vi "Read FP Control.vi"(8 "error in (no error)":errorcluster, 10 "Control Name":string="Configuration", 11 "Measure Object in":refnum<class "Measure Object.lvclass">) -> (0 "error out":errorcluster, 2 "Control Value":variant, 3 "Measure Object out":refnum<class "Measure Object.lvclass">)   [LabVIEW 2015, in "Measure Object.lvclass"]
uses:
  Measure Object.lvclass
  Measure Object.lvclass/Measure Object.ctl
  Read Front Panel ref.vi
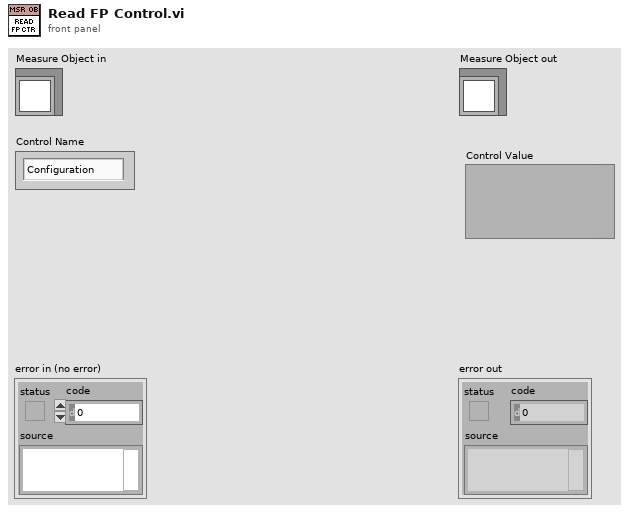
[diagram p1: front panel]
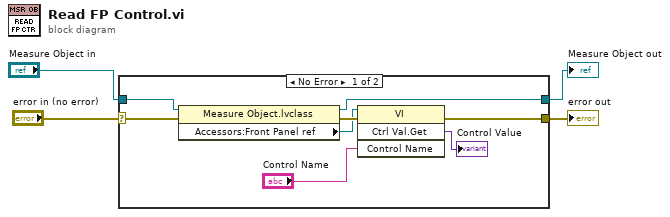
[diagram p0: block diagram]
diagram:
  n1 = case shown="No Error" "error in (no error)" {
    selector: "error in (no error)" -> [w9 w14]
    tunnel: [w6 w14] -> w3
    tunnel: [w7 w13] -> w1
    tunnel: "Measure Object in" -> [w8 w13]
    frame No Error {
      n2 = property class="Measure Object.lvclass"(reference=w8, error in=w9) -> (reference out=w7:refnum<class "Measure Object.lvclass">, error out=w12:errorcluster, "Accessors:Front Panel ref"=w5:refnum<vi>)
      n3 = invoke class="VI" method="Ctrl Val.Get"(reference=w5, error in=w12, "Control Name"="Control Name") -> (error out=w6:errorcluster, "Get Control Value Variant"=→"Control Value":variant)  [unwired: 1 in, 2 out]
    }
    frame Error {
    }
  }
  "error out" <- w3
  "Measure Object out" <- w1
